vi "Set_I16.vi"(8 "error in (no error)":errorcluster, 9 "value":i16=14, 10 "offset":i32, 11 "handle":i32) -> (0 "error out":errorcluster, 2 "error code":i32, 3 "tag handle out":i32)   [LabVIEW 2016]
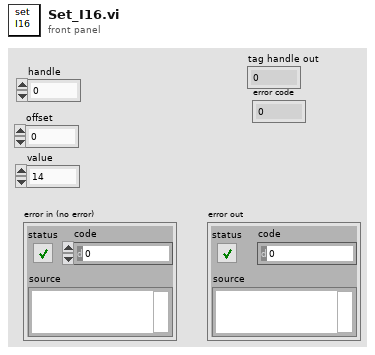
[diagram p1: front panel]
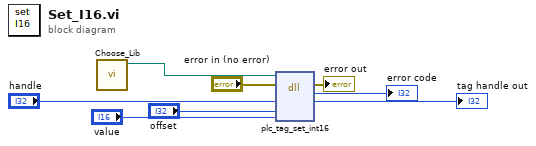
[diagram p0: block diagram]
diagram:
  n1 = call "Choose_Lib.vi"() -> ("appended path"=w1:path)  [unwired: 11 in]
  n2 = dll-call lib="home/dbowden/Desktop/libplctag-master/build/bin_dist/libplctag.so" fn="plc_tag_set_int16"(path in=w1, error in="error in (no error)", "tag handle"="handle", "offset"="offset", "value"="value") -> (error out=→"error out":errorcluster, "error code"=→"error code":i32, "tag handle"=→"tag handle out":i32)  [unwired: 3 in, 1 out]
